vi "Histogram Autoscale.vi"(7 "X Values":dbl[](array[numeric]), 9 "Histogram: h(x)":i32[](array[numeric])) -> (0 "Scale Min":dbl, 3 "Scale Max":dbl)   [LabVIEW 2018, in "Viewer.lvlib" / "Viewer.lvclass"]
uses:
  Viewer.lvclass
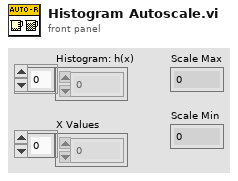
[diagram p1: front panel]
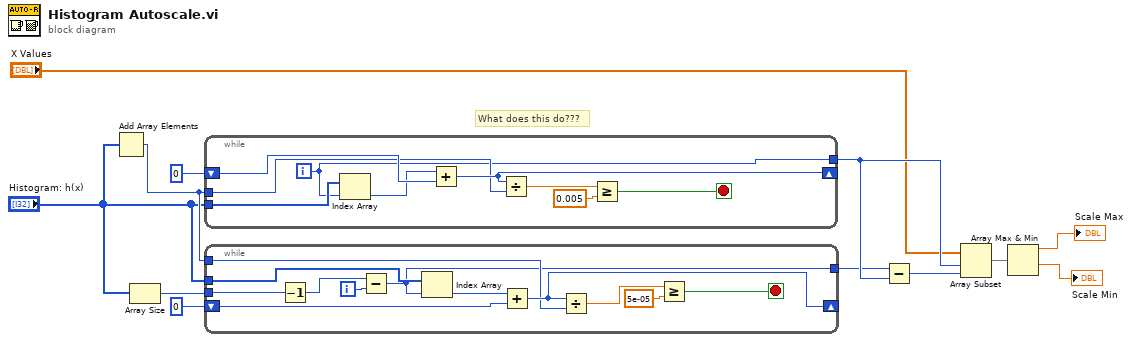
[diagram p0: block diagram]
diagram:
  # "What does this do???"
  n1 = Add Array Elements(numeric array="Histogram: h(x)") -> (sum=w8:i32)
  n2 = Array Size(array="Histogram: h(x)") -> (size(s)=w2:i32)
  n3 = while {
    tunnel: "Histogram: h(x)" -> [w20]
    shift-right: [w18] -> _
    shift-left: 0 -> [w21]
    tunnel: w8 -> [w17]
    tunnel: [w14] -> w5
    i -> [w14]
    stop <- w15 stop-if-true
    n4 = Index Array(array=w20, index=w14) -> (element=w19:i32)
    n5 = Add(x=w19, y=w21) -> (x+y=w18:i32)
    n6 = Divide(x=w18, y=w17) -> (x/y=w16:dbl)
    n7 = Greater Or Equal?(x=w16, y=0.005) -> (x >= y?=w15:bool)
  }
  n8 = while {
    tunnel: "Histogram: h(x)" -> [w32]
    shift-right: [w30] -> _
    shift-left: 0 -> [w33]
    tunnel: w8 -> [w29]
    tunnel: w2 -> [w25]
    tunnel: [w22] -> w4
    i -> [w23]
    stop <- w26 stop-if-true
    n9 = Decrement(x=w25) -> (x-1=w24:i32)
    n10 = Subtract(x=w24, y=w23) -> (x-y=w22:i32)
    n11 = Index Array(array=w32, index=w22) -> (element=w31:i32)
    n12 = Add(x=w31, y=w33) -> (x+y=w30:i32)
    n13 = Divide(x=w30, y=w29) -> (x/y=w28:dbl)
    n14 = Greater Or Equal?(x=w28, y=5e-05) -> (x >= y?=w26:bool)
  }
  n15 = Subtract(x=w4, y=w5) -> (x-y=w6:i32)
  n16 = Array Subset(array="X Values", index=w5, length=w6) -> (w7:dbl[])
  n17 = Array Max & Min(array=w7) -> (max value=→"Scale Max":dbl, min value=→"Scale Min":dbl)  [unwired: 2 out]
